vi "VI Server Test.vi"() -> ()   [LabVIEW 2009]
panel:
  out "error out":errorcluster
  in  "port number or service name (3363)":u16=3363
  in  "machine name (\"\":  open local reference)":string="127.0.0.1"
  out "Version Number 2":u32=134250501 format="%.0x"
  out "Get VI Version":string="8.0"
  out "Get VI Editor Version":string="8.0"
  in  "VI Path":path=path "C:/Users/PansinoSoft/Desktop/vi-snippet/L0004/VERSION INFO/8.0.vi"
  out "Version Number":u32=134250501 format="%.0x"
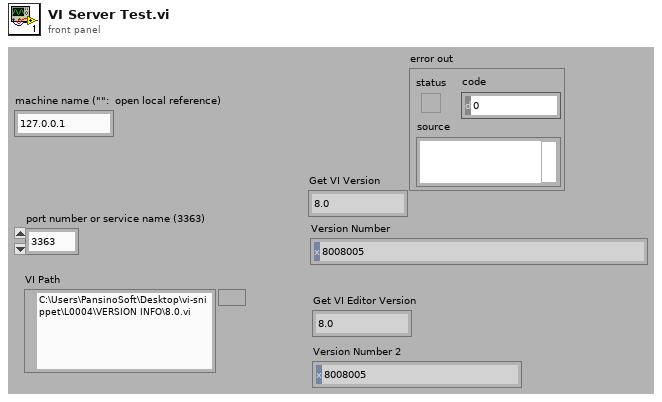
[diagram p1: front panel]
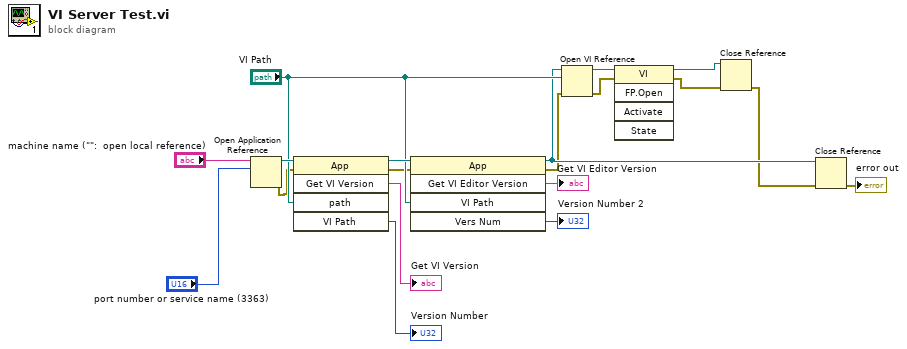
[diagram p0: block diagram]
diagram:
  n1 = Open Application Reference(10:"port number or service name (3363)", 11:"machine name (\"\":  open local reference)") -> (0:w9:errorcluster, 3:w19:refnum<vi>)  [unwired: 2 in]
  n2 = invoke class="App" method="Get VI Version"(reference=w19, error in=w9, "path"="VI Path") -> (reference out=w14:refnum<vi>, error out=w8:errorcluster, "GetVIVers"=→"Get VI Version":string, "VI Path"=→"Version Number":u32)  [unwired: 2 in, 1 out]
  n3 = invoke class="App" method="Get VI Editor Version"(reference=w14, error in=w8, "VI Path"="VI Path") -> (reference out=w10:refnum<vi>, error out=w7:errorcluster, "Get VI Editor Version"=→"Get VI Editor Version":string, "Vers Num"=→"Version Number 2":u32)  [unwired: 2 in, 1 out]
  n4 = Open VI Reference(application reference (local)=w10, vi path="VI Path", error in (no error)=w7) -> (vi reference=w12:refnum<vi>, error out=w6:errorcluster)  [unwired: 3 in]
  n5 = invoke class="VI" method="FP.Open"(reference=w12, error in=w6) -> (reference out=w11:refnum<vi>, error out=w5:errorcluster)  [unwired: 3 in, 3 out]
  n6 = Close Reference(reference=w11, error in (no error)=w5) -> (error out=w4:errorcluster)
  n7 = Close Reference(reference=w10, error in (no error)=w4) -> (error out=→"error out":errorcluster)
